vi "Main.vi"() -> ()   [LabVIEW 2014]
uses:
  Enum State Typedef.ctl
  <vilib>/_DAQmxBase/Internals/DAQmxBase Create Channel (AI-Voltage-Basic).vi
  <vilib>/_DAQmxBase/Internals/DAQmxBase Timing (Sample Clock).vi
  <vilib>/_DAQmxBase/Internals/DAQmxBase Read (Analog 2D DBL NChan NSamp).vi
  <vilib>/Utility/error.llb/DialogType.ctl
  <vilib>/Utility/file.llb/Write To Spreadsheet File (DBL).vi
  <vilib>/Utility/file.llb/Write To Spreadsheet File (string).vi
  <vilib>/Utility/file.llb/Write To Spreadsheet File (I64).vi
panel:
  in  "Amount of Time per Recording (seconds)":dbl
  in  "Sample Rate":i32=1000
  in  "physical channels":tag
  in  "Stop Button":bool
  out "Waveform Graph":waveform(dbl)(graph)
  in  "High Pass Filter":enum16{""}(ring)
  in  "Low Pass Filter":enum16{""}(ring)
  in  "Gain":enum16{""}(ring)
  in  "Notch Filter":bool
  in  "Amplifier Model":u16(ring) items=["Select a Model", "AM 1700", "BMA 200"]
  in  "AC/DC Switch":bool
  in  "Temperature (deg C)":dbl
  in  "User Comments":string
  in  "Start Time hr/min":string
  in  "Date mm/dd/yy":string
  in  "Species":string
  in  "Exit Button":bool
  in  "Record Button":bool
  # "Do a length of recording"
  # "Must enter numbers into here before you run"
  # "DC"
  # "AC"
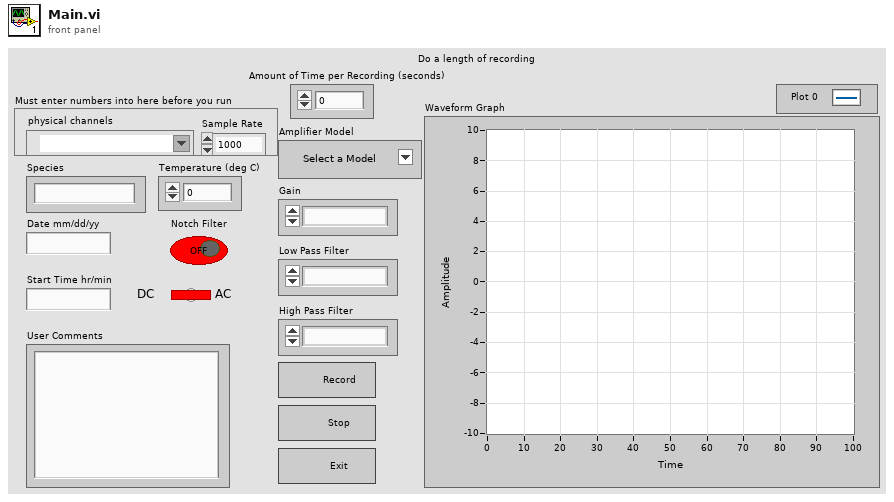
[diagram p1: front panel]
types:
  T1 = typedef "Enum State Typedef.ctl" = enum16{"", "Stop", "Exit", "Record", "Create File"}
  T2 = cluster{"Notch Filter":bool, "AC/DC Switch":bool}
  T3 = typedef "DialogType.ctl" = u16
  T4 = cluster{"Species":string, "Date mm/dd/yy":string, "Start Time hr/min":string, "User Comments":string}
  T5 = cluster{"Gain":enum16{""}, "Low Pass Filter":enum16{""}, "High Pass Filter":enum16{""}}
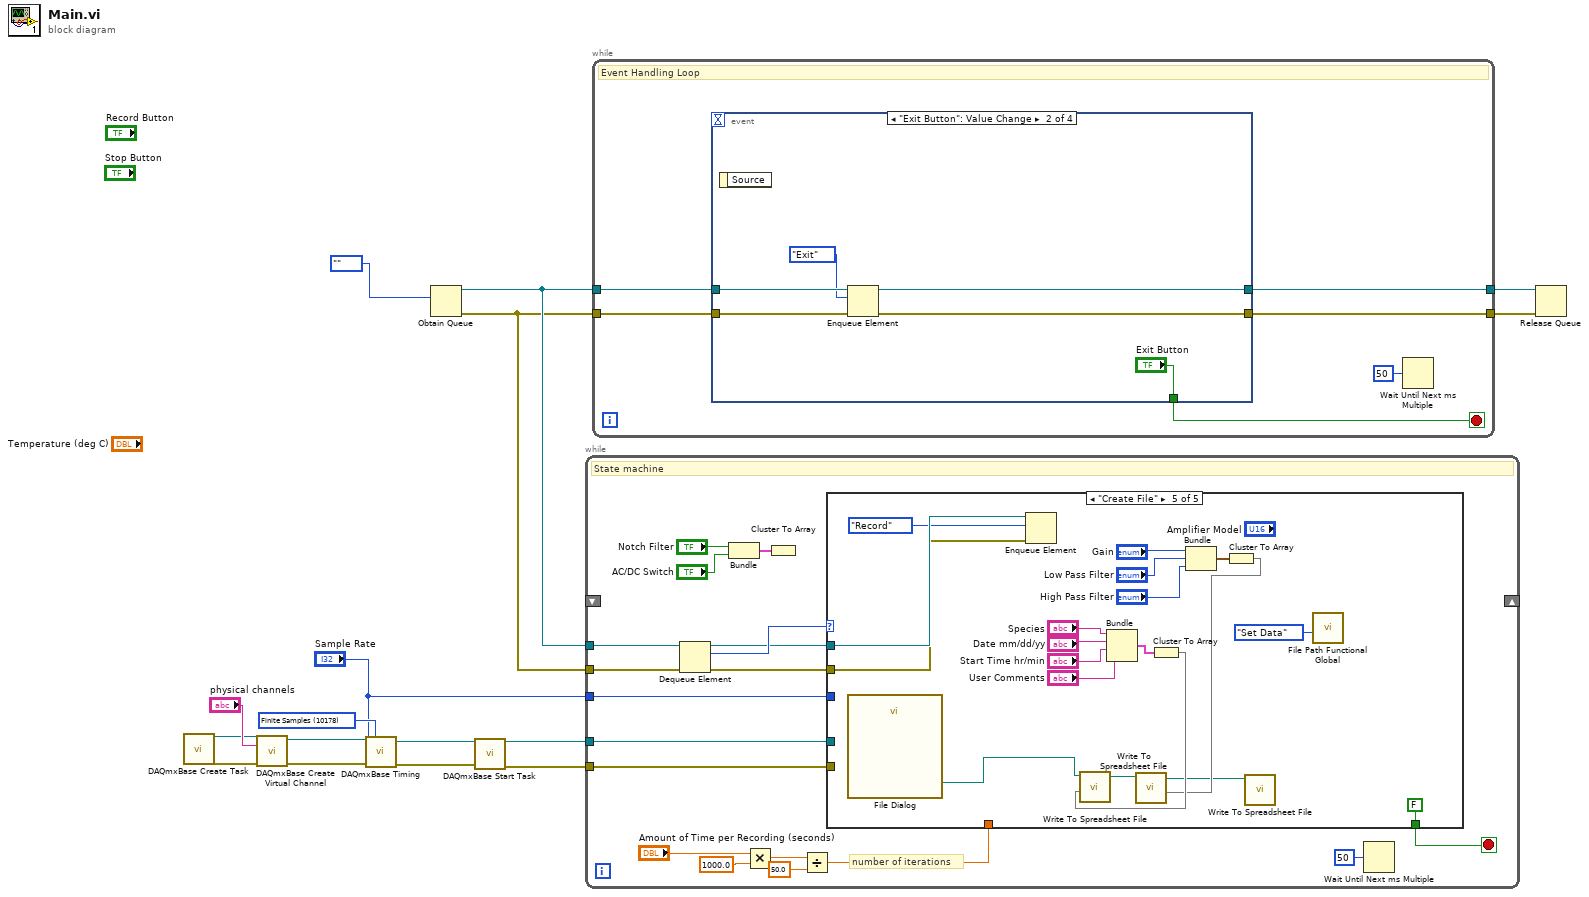
[diagram p0: block diagram]
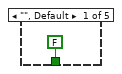
[diagram p2: hidden frame]
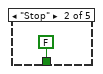
[diagram p3: hidden frame]
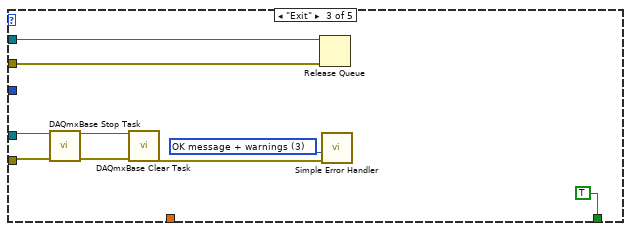
[diagram p4: hidden frame]
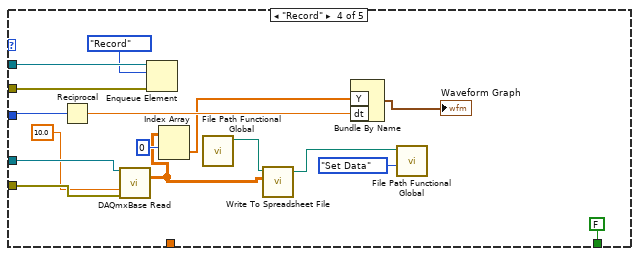
[diagram p5: hidden frame]
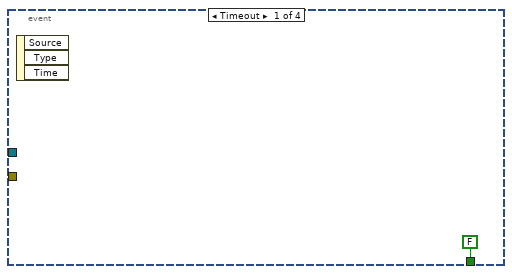
[diagram p6: hidden frame]
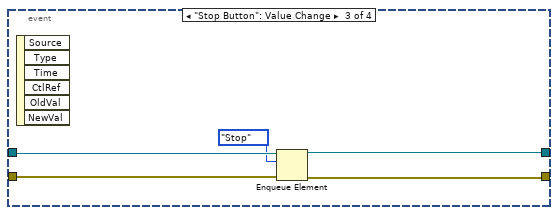
[diagram p7: hidden frame]
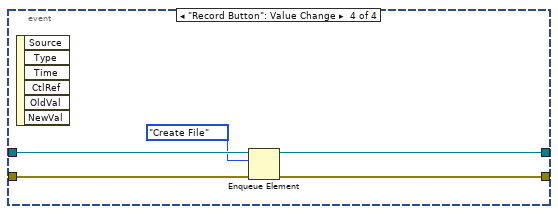
[diagram p8: hidden frame]
diagram:
  w6 = 10178 items=["Finite Samples"=10178, "Continuous Samples"=10123, "Hardware Timed Single Point"=12522] ("sample mode")
  n1 = call <vilib>:"DAQmxBase Create Task.vi"() -> ("task out"=w10:refnum<k21>, "error out"=w9:errorcluster)  [unwired: 14 in]
  n2 = call-poly <vilib>:"DAQmxBase Create Virtual Channel.vi"("task in"=w10, "physical channels"="physical channels", "error in"=w9) -> ("task out"=w8:refnum<k21>, "error out"=w7:errorcluster)  [unwired: 11 in]
  n3 = call-poly <vilib>:"DAQmxBase Timing.vi"("task/channels in"=w8, "sample mode"=w6, "rate"="Sample Rate", "error in"=w7) -> ("task out"=w5:refnum<k21>, "error out"=w4:errorcluster)  [unwired: 10 in]
  n4 = Obtain Queue(element data type=Enum_State_Typedef."" ("State")) -> (queue out=w13:refnum<queue>, error out=w12:errorcluster)  [unwired: 4 in, 1 out]
  n5 = call <vilib>:"DAQmxBase Start Task.vi"("task/channels in"=w5, "error in"=w4) -> ("task out"=w2:refnum<k21>, "error out"=w3:errorcluster)  [unwired: 12 in]
  n6 = while {
    tunnel: w13 -> [w34]
    tunnel: w12 -> [w33]
    tunnel: w3 -> [w27]
    tunnel: w2 -> [w28]
    tunnel: "Sample Rate" -> [w26]
    shift-right: _ -> [_]
    shift-left: _ -> [_]
    stop <- w31 stop-if-true
    # "number of iterations"
    # "State machine"
    n7 = Dequeue Element(queue=w34, error in (no error)=w33) -> (queue out=w30:refnum<queue>, element=w32:T1, error out=w29:errorcluster)  [unwired: 1 in, 1 out]
    n8 = Bundle("Notch Filter"="Notch Filter", "AC/DC Switch"="AC/DC Switch") -> (w25:T2)  [unwired: 1 in]
    n9 = Multiply(x="Amount of Time per Recording (seconds)", y=1000.0) -> (x*y=w19:dbl)
    n10 = Cluster To Array(cluster=w25) -> ()  [unwired: 1 out]
    n11 = Divide(x=w19, y=50.0) -> (x/y=w17:dbl)
    n12 = case shown="\"Create File\"" w32 {
      tunnel: [FALSE FALSE TRUE FALSE FALSE] -> w31
      tunnel: w30 -> [_ _ w38 w60 w79]
      tunnel: w29 -> [_ _ w37 w59 w78]
      tunnel: w28 -> [_ _ w42 w57 _]
      tunnel: w27 -> [_ _ w41 w56 _]
      tunnel: w26 -> [_ _ _ w51 _]
      tunnel: w17 -> [_ _ _ _ _]
      frame "", Default {
      }
      frame "Stop" {
      }
      frame "Exit" {
        w39 = T3 3 items=["no dialog", "OK message", "continue or stop message", "OK message + warnings", "continue/stop + warnings"] ("type of dialog (OK msg:1)")
        n13 = call <vilib>:"DAQmxBase Stop Task.vi"("task/channels in"=w42, "error in"=w41) -> ("task out"=w44:refnum<k21>, "error out"=w43:errorcluster)  [unwired: 12 in]
        n14 = call <vilib>:"DAQmxBase Clear Task.vi"("task in"=w44, "error in"=w43) -> ("error out"=w40:errorcluster)  [unwired: 13 in]
        n15 = Release Queue(queue=w38, error in (no error)=w37) -> ()  [unwired: 1 in, 3 out]
        n16 = call <vilib>:"Simple Error Handler.vi"("type of dialog (OK msg:1)"=w39, "error in (no error)"=w40) -> ()  [unwired: 3 in, 5 out]
      }
      frame "Record" {
        n17 = Reciprocal(x=w51) -> (1/x=w50:dbl)
        n18 = call-poly <vilib>:"DAQmxBase Read.vi"("task/channels in"=w57, "timeout"=10.0, "error in"=w56) -> ("data"=w46:dbl[][])  [unwired: 10 in, 2 out]
        n19 = Enqueue Element(queue=w60, element=Enum_State_Typedef."Record", error in (no error)=w59) -> ()  [unwired: 1 in, 3 out]
        n20 = Index Array(array=w46, index (row)=0) -> (element=w47:dbl[])  [unwired: 1 in]
        n21 = call "File Path Functional Global.vi"() -> ("File Path Output"=w54:path)  [unwired: 11 in]
        n22 = call-poly <vilib>:"Write To Spreadsheet File.vi"("2D data"=w46, "file path (dialog if empty)"=w54) -> ("new file path (Not A Path if cancelled)"=w52:path)  [unwired: 6 in]
        n23 = Bundle By Name("Y"=w47, "dt"=w50) -> (→"Waveform Graph":waveform(dbl))  [unwired: 1 in]
        n24 = call "File Path Functional Global.vi"("Enum"=enum16{"Get Data", "Set Data"}."Set Data", "File Path Control"=w52) -> ()  [unwired: 9 in, 1 out]
      }
      frame "Create File" {
        n25 = call "File Dialog"() -> ("selected path"=w69:path)  [unwired: 12 in, 3 out]
        n26 = Enqueue Element(queue=w79, element=Enum_State_Typedef."Record", error in (no error)=w78) -> ()  [unwired: 1 in, 3 out]
        n27 = Bundle("Species"="Species", "Date mm/dd/yy"="Date mm/dd/yy", "Start Time hr/min"="Start Time hr/min", "User Comments"="User Comments") -> (w72:T4)  [unwired: 1 in]
        n28 = Cluster To Array(cluster=w72) -> (array=w71:string[])
        n29 = call-poly <vilib>:"Write To Spreadsheet File.vi"("1D data"=w71, "file path (dialog if empty)"=w69) -> ("new file path (Not A Path if cancelled)"=w63:path)  [unwired: 6 in]
        n30 = Bundle("Gain"="Gain", "Low Pass Filter"="Low Pass Filter", "High Pass Filter"="High Pass Filter") -> (w68:T5)  [unwired: 1 in]
        n31 = Cluster To Array(cluster=w68) -> (array=w64:enum16{""}[])
        n32 = call-poly <vilib>:"Write To Spreadsheet File.vi"("1D data"=w64, "file path (dialog if empty)"=w63) -> ("new file path (Not A Path if cancelled)"=w62:path)  [unwired: 6 in]
        n33 = call-poly <vilib>:"Write To Spreadsheet File.vi"("file path (dialog if empty)"=w62) -> ()  [unwired: 7 in, 1 out]
        n34 = call "File Path Functional Global.vi"("Enum"=enum16{"Get Data", "Set Data"}."Set Data") -> ()  [unwired: 10 in, 1 out]
      }
    }
    n35 = Wait Until Next ms Multiple(millisecond multiple=u32 50) -> ()  [unwired: 1 out]
  }
  n36 = while {
    tunnel: w13 -> [w85]
    tunnel: w12 -> [w84]
    tunnel: [w83] -> w15
    tunnel: [w82] -> w14
    stop <- w86 stop-if-true
    # "Event Handling Loop"
    n37 = event shown="[1] \"Exit Button\": Value Change" {
      selector: _ -> [_ _ _ _]
      dyn-events: _ -> [_ _ _ _]
      timeout: _ -> [_ _ _ _]
      tunnel: [FALSE ("Exit Button") "Exit Button" _ _] -> w86
      tunnel: w85 -> [_ w92 w98 w103]
      tunnel: w84 -> [_ w91 w97 w102]
      tunnel: [_ w90 w95 w100] -> w83
      tunnel: [_ w89 w96 w101] -> w82
      event Timeout {
        n38 = event-data() -> ()  [unwired: 1 in, 3 out]
      }
      event "Exit Button": Value Change {
        n39 = event-data() -> ()  [unwired: 1 in, 1 out]
        n40 = Enqueue Element(queue=w92, element=Enum_State_Typedef."Exit", error in (no error)=w91) -> (queue out=w90:refnum<queue>, error out=w89:errorcluster)  [unwired: 1 in, 1 out]
      }
      event "Stop Button": Value Change {
        n41 = event-data() -> ()  [unwired: 1 in, 6 out]
        n42 = Enqueue Element(queue=w98, element=Enum_State_Typedef."Stop", error in (no error)=w97) -> (queue out=w95:refnum<queue>, error out=w96:errorcluster)  [unwired: 1 in, 1 out]
      }
      event "Record Button": Value Change {
        n43 = event-data() -> ()  [unwired: 1 in, 6 out]
        n44 = Enqueue Element(queue=w103, element=Enum_State_Typedef."Create File", error in (no error)=w102) -> (queue out=w100:refnum<queue>, error out=w101:errorcluster)  [unwired: 1 in, 1 out]
      }
    }
    n45 = Wait Until Next ms Multiple(millisecond multiple=u32 50) -> ()  [unwired: 1 out]
  }
  n46 = Release Queue(queue=w15, error in (no error)=w14) -> ()  [unwired: 1 in, 3 out]
